vi "Run Instruction.vi"(8 "error in (no error)":errorcluster, 10 "ROM":bool[][](array[boolean]), 11 "TD4 in":refnum<class "TD4.lvclass">) -> (0 "error out":errorcluster, 3 "TD4 out":refnum<class "TD4.lvclass">)   [LabVIEW 2025, in "TD4.lvclass"]
uses:
  TD4.lvclass
  TD4.lvclass/TD4.ctl
  Add with Carry.vi
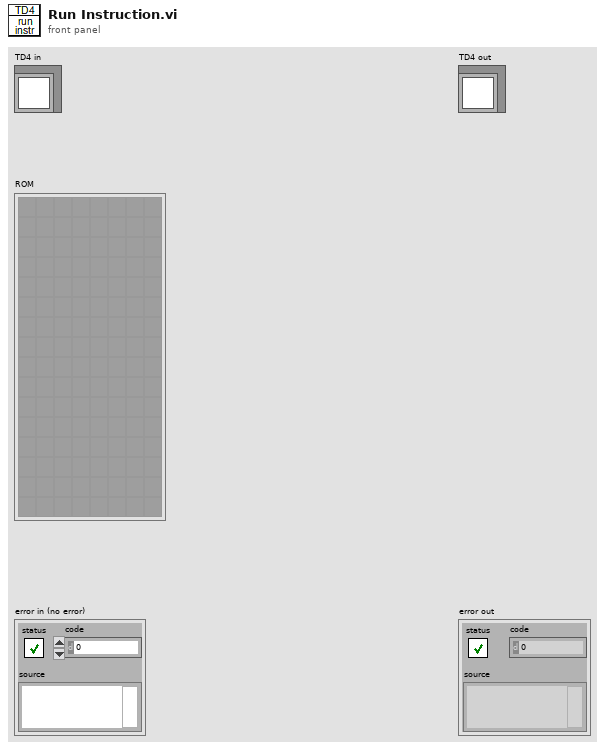
[diagram p1: front panel]
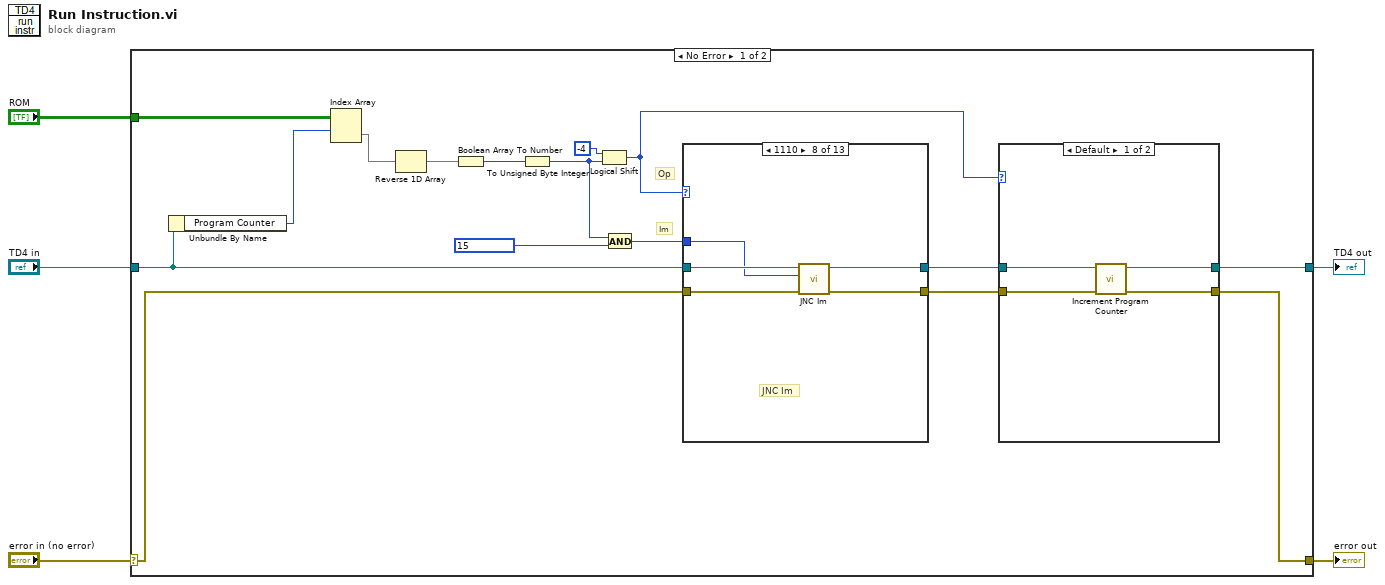
[diagram p0: block diagram]
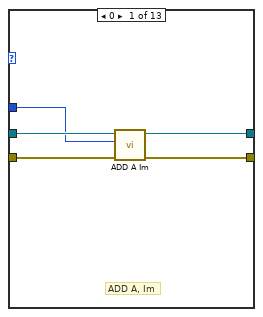
[diagram p3: hidden frame]
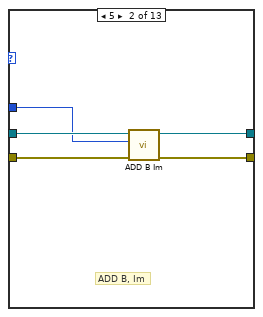
[diagram p4: hidden frame]
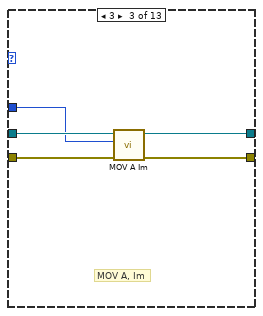
[diagram p5: hidden frame]
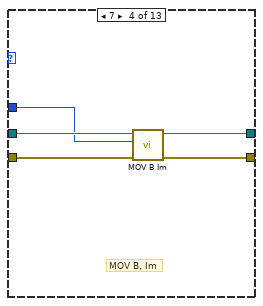
[diagram p6: hidden frame]
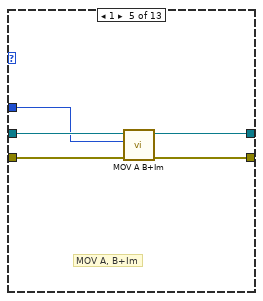
[diagram p7: hidden frame]
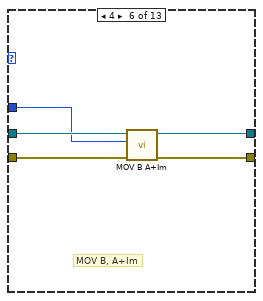
[diagram p8: hidden frame]
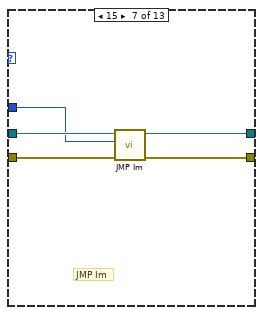
[diagram p9: hidden frame]
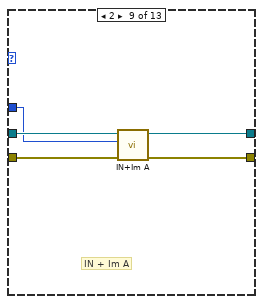
[diagram p10: hidden frame]
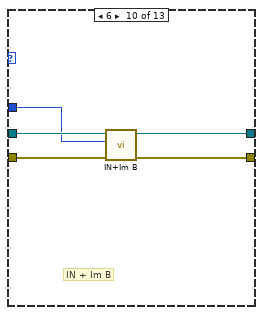
[diagram p11: hidden frame]
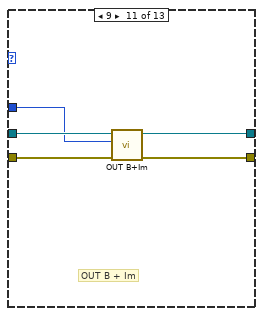
[diagram p12: hidden frame]
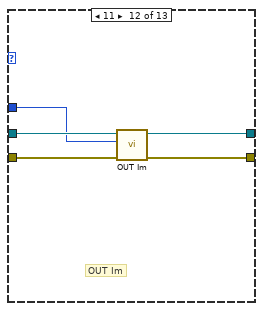
[diagram p13: hidden frame]
diagram:
  n1 = case shown="No Error" "error in (no error)" {
    selector: "error in (no error)" -> [w13 w90]
    tunnel: [w7 w90] -> w4
    tunnel: [w9 w91] -> w2
    tunnel: "TD4 in" -> [w19 w91]
    tunnel: "ROM" -> [w21 _]
    frame No Error {
      # "Op"
      # "Im"
      n2 = Unbundle By Name(w19) -> ("Program Counter"=w20:u8)
      n3 = Index Array(array=w21, index (row)=w20) -> (element=w16:bool[])  [unwired: 1 in]
      n4 = Reverse 1D Array(array=w16) -> (reversed array=w17:bool[])
      n5 = Boolean Array To Number(Boolean array=w17) -> (number=w12:u32)
      n6 = To Unsigned Byte Integer(number=w12) -> (unsigned 8bit integer=w11:u8)
      n7 = Logical Shift(y=i16 -4, x=w11) -> (x << y=w10:u8)
      n8 = And(x=w11, y=u8 15) -> (x .and. y?=w14:u8)
      n9 = case shown="1110" w10 {
        tunnel: w19 -> [w32 w37 w42 w47 w52 w54 w62 w65 w72 w77 w82 w87 w89]
        tunnel: [w31 w36 w41 w46 w50 w57 w61 w67 w71 w76 w81 w86 w89] -> w8
        tunnel: w14 -> [w28 w33 w38 w43 w51 w53 w58 w63 w68 w73 w78 w83 _]
        tunnel: w13 -> [w30 w34 w39 w44 w48 w55 w59 w64 w69 w74 w79 w84 w88]
        tunnel: [w29 w35 w40 w45 w49 w56 w60 w66 w70 w75 w80 w85 w88] -> w6
        frame 0 {
          # "ADD A, Im"
          n10 = call "ADD A Im.vi"("error in (no error)"=w30, "Im"=w28, "TD4 in"=w32) -> ("error out"=w29:errorcluster, "TD4 out"=w31:refnum<class "TD4.lvclass">)  [unwired: 7 in]
        }
        frame 5 {
          # "ADD B, Im"
          n11 = call "ADD B Im.vi"("error in (no error)"=w34, "Im"=w33, "TD4 in"=w37) -> ("error out"=w35:errorcluster, "TD4 out"=w36:refnum<class "TD4.lvclass">)  [unwired: 7 in]
        }
        frame 3 {
          # "MOV A, Im"
          n12 = call "MOV A Im.vi"("error in (no error)"=w39, "Im"=w38, "TD4 in"=w42) -> ("error out"=w40:errorcluster, "TD4 out"=w41:refnum<class "TD4.lvclass">)  [unwired: 7 in]
        }
        frame 7 {
          # "MOV B, Im"
          n13 = call "MOV B Im.vi"("error in (no error)"=w44, "Im"=w43, "TD4 in"=w47) -> ("error out"=w45:errorcluster, "TD4 out"=w46:refnum<class "TD4.lvclass">)  [unwired: 7 in]
        }
        frame 1 {
          # "MOV A, B+Im"
          n14 = call "MOV A B+Im.vi"("error in (no error)"=w48, "Im"=w51, "TD4 in"=w52) -> ("error out"=w49:errorcluster, "TD4 out"=w50:refnum<class "TD4.lvclass">)  [unwired: 7 in]
        }
        frame 4 {
          # "MOV B, A+Im"
          n15 = call "MOV B A+Im.vi"("error in (no error)"=w55, "Im"=w53, "TD4 in"=w54) -> ("error out"=w56:errorcluster, "TD4 out"=w57:refnum<class "TD4.lvclass">)  [unwired: 7 in]
        }
        frame 15 {
          # "JMP Im"
          n16 = call "JMP Im.vi"("error in (no error)"=w59, "Im"=w58, "TD4 in"=w62) -> ("error out"=w60:errorcluster, "TD4 out"=w61:refnum<class "TD4.lvclass">)  [unwired: 7 in]
        }
        frame 14 {
          # "JNC Im"
          n17 = call "JNC Im.vi"("error in (no error)"=w64, "Im"=w63, "TD4 in"=w65) -> ("error out"=w66:errorcluster, "TD4 out"=w67:refnum<class "TD4.lvclass">)  [unwired: 7 in]
        }
        frame 2 {
          # "IN + Im A"
          n18 = call "IN+Im A.vi"("error in (no error)"=w69, "Im"=w68, "TD4 in"=w72) -> ("error out"=w70:errorcluster, "TD4 out"=w71:refnum<class "TD4.lvclass">)  [unwired: 7 in]
        }
        frame 6 {
          # "IN + Im B"
          n19 = call "IN+Im B.vi"("error in (no error)"=w74, "Im"=w73, "TD4 in"=w77) -> ("error out"=w75:errorcluster, "TD4 out"=w76:refnum<class "TD4.lvclass">)  [unwired: 7 in]
        }
        frame 9 {
          # "OUT B + Im"
          n20 = call "OUT B+Im.vi"("error in (no error)"=w79, "Im"=w78, "TD4 in"=w82) -> ("error out"=w80:errorcluster, "TD4 out"=w81:refnum<class "TD4.lvclass">)  [unwired: 7 in]
        }
        frame 11 {
          # "OUT Im"
          n21 = call "OUT Im.vi"("error in (no error)"=w84, "Im"=w83, "TD4 in"=w87) -> ("error out"=w85:errorcluster, "TD4 out"=w86:refnum<class "TD4.lvclass">)  [unwired: 7 in]
        }
        frame Default {
          # "Do nothing is opcode is otherwise"
        }
      }
      n22 = case shown="Default" w10 {
        tunnel: [w24 w27] -> w9
        tunnel: w8 -> [w25 w27]
        tunnel: [w23 w26] -> w7
        tunnel: w6 -> [w22 w26]
        frame Default {
          n23 = call "Increment Program Counter.vi"("error in (no error)"=w22, "TD4 in"=w25) -> ("error out"=w23:errorcluster, "TD4 out"=w24:refnum<class "TD4.lvclass">)  [unwired: 8 in]
        }
        frame 14, 15 {
          # "Don't increment Program Counter\nfor JMP and JNC opcodes"
        }
      }
    }
    frame Error {
    }
  }
  "error out" <- w4
  "TD4 out" <- w2
